vi "interpolate.vi"() -> ()   [LabVIEW 2024]
uses:
  <vilib>/Analysis/baseanly.llb/Mean (DBL).vi
  <vilib>/Analysis/NI_AALPro.lvlib
  <vilib>/Analysis/NI_AALBase.lvlib
panel:
  out "f(0)":dbl[](array[numeric]) format="%#_3g"
  out "means":dbl[](array[numeric]) format="%#_3g"
  out "div":dbl[][](array[numeric]) format="%#_3g"
  in  "WidthY":dbl[](array[numeric])=[207.0, 462.0]
  in  "PositionY":dbl[](array[numeric])=[145.0, 330.0]
  in  "X":dbl[](array[numeric])=[411.4, 914.3]
  out "XY Graph":cluster{dbl[], dbl[]}[](graph)
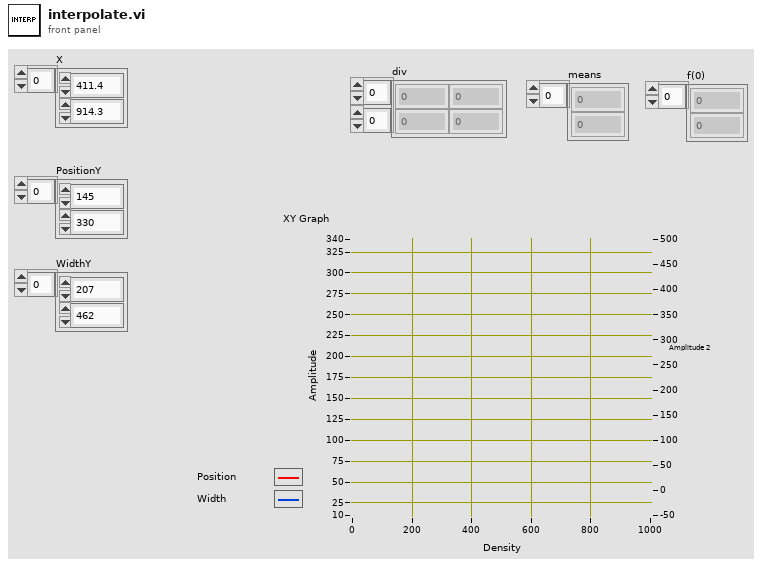
[diagram p1: front panel]
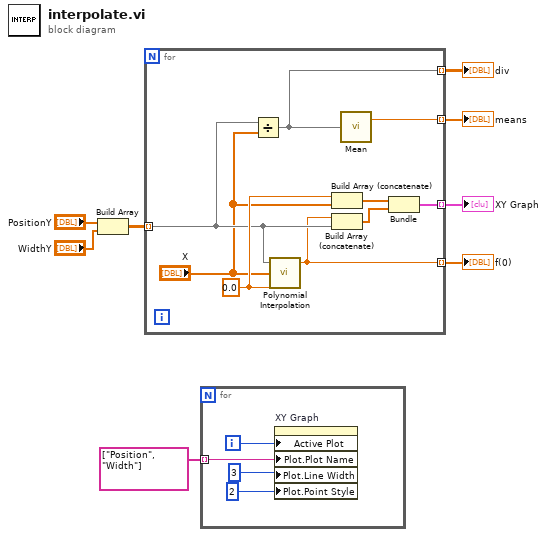
[diagram p0: block diagram]
diagram:
  n1 = Build Array("PositionY", "WidthY") -> (w6:dbl[][])
  n2 = for {
    tunnel: [w16] -> w8 mode=indexing
    tunnel: w6 -> [w13] mode=indexing
    tunnel: [w11] -> w4 mode=indexing
    tunnel: [w10] -> w3 mode=indexing
    tunnel: [w9] -> w2 mode=indexing
    w14 = 0.0 ("x value")
    n3 = Divide(x=w13, y="X") -> (x/y=w11:dbl[])
    n4 = call <vilib>:"Polynomial Interpolation.vi"("x value"=w14, "X"="X", "Y"=w13) -> ("interpolation value"=w9:dbl)  [unwired: 2 out]
    n5 = Build Array (concatenate)(w14, "X") -> (w17:dbl[])
    n6 = Build Array (concatenate)(w9, w13) -> (w15:dbl[])
    n7 = call-poly <vilib>:"Mean.vi"("X"=w11) -> ("mean"=w10:dbl)  [unwired: 1 out]
    n8 = Bundle(w17, w15) -> (w16:cluster{dbl[], dbl[]})  [unwired: 1 in]
  }
  "XY Graph" <- w8
  "div" <- w4
  "means" <- w3
  "f(0)" <- w2
  n9 = for {
    tunnel: string[] ["Position", "Width"] ("array type (2D Dbl)") -> [w20] mode=indexing
    i -> [w21]
    n10 = property on="XY Graph" class="XYGraph (strict)"("Active Plot"=w21, "Plot.Plot Name"=w20, "Plot.Line Width"=u8 3, "Plot.Point Style"=u8 2) -> ()  [unwired: 2 in, 2 out]
  }
